vi "ReadAllGlobalsALB.vi"() -> (0 "J1 buttons":T6, 1 "Axes out":T3 {"Slider" format="%#_4g"; "Axis 2" format="%#_4g"; "Axis 1" format="%#_4g"; "Axis 0" format="%#_4g"}, 2 "Sol out":T8, 3 "AI out":T7, 4 "J2 buttons":T5, 5 "Gyro_Data":T2, 6 "Axes out 2":T1 {"Switch" format="%#_4g"; "Axis 2" format="%#_4g"; "Axis 1" format="%#_4g"; "Axis 0" format="%#_4g"}, 8 "DI out":T4)   [LabVIEW 2017]
uses:
  CtrlRefs/SolenoidsDisplayALB.ctl
  CtrlRefs/AnalogDisplayALB.ctl
  CtrlRefs/JoyStick1ALB.ctl
  CtrlRefs/JoyStick2ALB.ctl
  CtrlRefs/DioDisplayALB.ctl
  CtrlRefs/JoyStick1ALV(Analog).ctl
  Support Code/Gyro/Gyro_TypeDef.ctl
  CtrlRefs/JoyStick2ALB(Analog).ctl
  Framework/Robot Global Data.vi
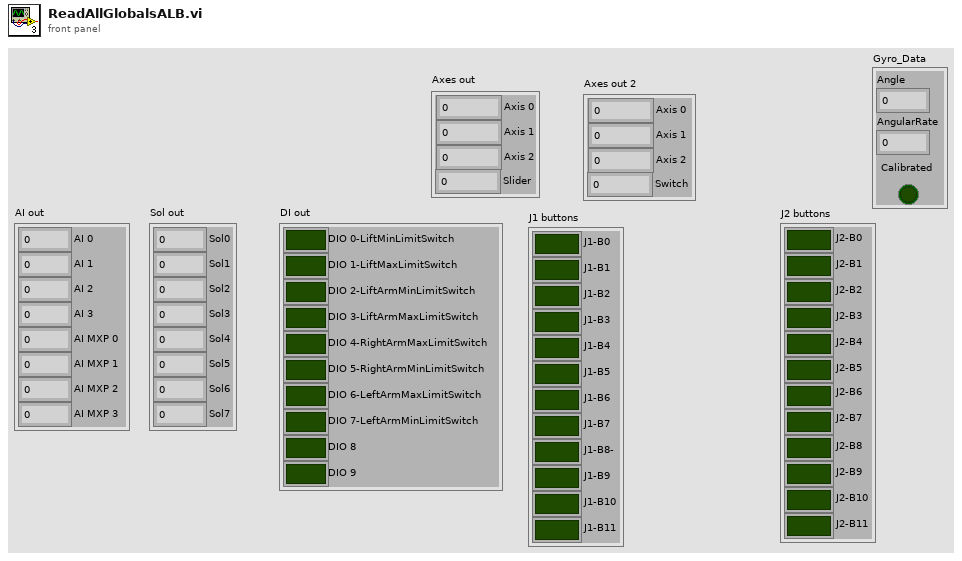
[diagram p1: front panel]
types:
  T1 = typedef "JoyStick2ALB(Analog).ctl" = cluster{"Axis 0":dbl, "Axis 1":dbl, "Axis 2":dbl, "Switch":dbl}
  T2 = typedef "Gyro_TypeDef.ctl" = cluster{"Angle":dbl, "AngularRate":dbl, "Calibrated":bool}
  T3 = typedef "JoyStick1ALV(Analog).ctl" = cluster{"Axis 0":dbl, "Axis 1":dbl, "Axis 2":dbl, "Slider":dbl}
  T4 = typedef "DioDisplayALB.ctl" = cluster{"DIO 0-LiftMinLimitSwitch":bool, "DIO 1-LiftMaxLimitSwitch":bool, "DIO 2-LiftArmMinLimitSwitch":bool, "DIO 3-LiftArmMaxLimitSwitch":bool, "DIO 4-RightArmMaxLimitSwitch":bool, "DIO 5-RightArmMinLimitSwitch":bool, "DIO 6-LeftArmMaxLimitSwitch":bool, "DIO 7-LeftArmMinLimitSwitch":bool, "DIO 8":bool, "DIO 9":bool}
  T5 = typedef "JoyStick2ALB.ctl" = cluster{"J2-B0":bool, "J2-B1":bool, "J2-B2":bool, "J2-B3":bool, "J2-B4":bool, "J2-B5":bool, "J2-B6":bool, "J2-B7":bool, "J2-B8":bool, "J2-B9":bool, "J2-B10":bool, "J2-B11":bool}
  T6 = typedef "JoyStick1ALB.ctl" = cluster{"J1-B0":bool, "J1-B1":bool, "J1-B2":bool, "J1-B3":bool, "J1-B4":bool, "J1-B5":bool, "J1-B6":bool, "J1-B7":bool, "J1-B8-":bool, "J1-B9":bool, "J1-B10":bool, "J1-B11":bool}
  T7 = typedef "AnalogDisplayALB.ctl" = cluster{"AI 0":dbl, "AI 1":dbl, "AI 2":dbl, "AI 3":dbl, "AI MXP 0":dbl, "AI MXP 1":dbl, "AI MXP 2":dbl, "AI MXP 3":dbl}
  T8 = typedef "SolenoidsDisplayALB.ctl" = cluster{"CanLift (0)":i32, "StackLift1 (1)":i32, "StackLift2 (2)":i32, "CanPosition (3)":i32, "CanLift4 (4)":i32, "CanLift (5)":i32, "Latch1 (6)":i32, "Latch2 (7)":i32}
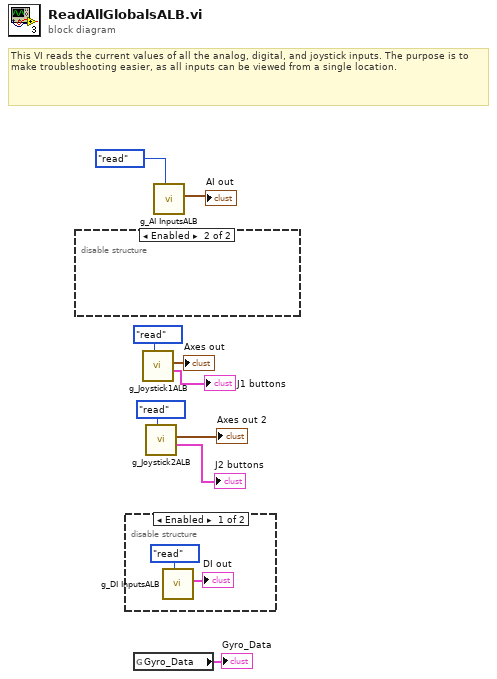
[diagram p0: block diagram]
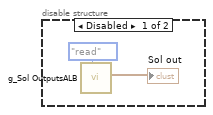
[diagram p3: hidden frame]
diagram:
  # "This VI reads the current values of all the analog, digital, and joystick inputs. The purpose is to make troubleshooting easier, as all inputs can be viewed from a single location."
  n1 = disable-structure shown="Enabled" {
    frame Disabled {
      n2 = call "g_Sol OutputsALB.vi"("Action"=enum16{"initialize", "read", "write"}."read") -> ("DI out"=→"Sol out":T8)  [unwired: 10 in]
    }
    frame Enabled {
    }
  }
  n3 = disable-structure shown="Enabled" {
    frame Enabled {
      n4 = call "g_DI InputsALB.vi"("Action"=enum16{"initialize", "read", "write"}."read") -> ("DI out"=→"DI out":T4)  [unwired: 10 in]
    }
    frame Disabled {
    }
  }
  n5 = global read "Robot Global Data.vi" "Gyro_Data"() -> (→"Gyro_Data":T2)
  n6 = call "g_Joystick1ALB.vi"("Action"=enum16{"initialize", "read", "write"}."read") -> ("Buttons out"=→"J1 buttons":T6, "Axes out"=→"Axes out":T3)  [unwired: 7 in, 2 out]
  n7 = call "g_Joystick2ALB.vi"("Action"=enum16{"initialize", "read", "write"}."read") -> ("Buttons out"=→"J2 buttons":T5, "Axes out"=→"Axes out 2":T1)  [unwired: 7 in, 2 out]
  n8 = call "g_AI InputsALB.vi"("Action"=enum16{"initialize", "read", "write"}."read") -> ("AI out"=→"AI out":T7)  [unwired: 10 in]
